vi "Stage Controller.vi"() -> ()   [LabVIEW 2013]
uses:
  <vilib>/Analysis/3filter.llb/Filter Passband Type.ctl
  <userlib>/Agilis Labview 7.1/AGILIS.llb/enter / leave remote mode.vi
  <vilib>/LabVIEW Hacker/LINX/Public/Peripherals/Analog/Analog Read 1 Chan.vi
  <vilib>/LabVIEW Hacker/LINX/LVH-LINX.lvlib
  <vilib>/ptbypt/NI_PtbyPt.lvlib
  <vilib>/Analysis/NI_AALBase.lvlib
panel:
  in  "Move Slide Back":bool
  in  "Move Slide":bool
  in  "Slide Jog Speed":i32(slide) scale=1.0..3.0
  in  "Tab Control":T1(tab)
  out "Main Sig":dbl[][](graph)
  out "Main Output":dbl(graph)
  in  "Arduino Serial Port":refnum<visa-resource-name>="COM3"
  out "Device Name":string
  in  "Analog Channel":u8
  out "Filtered Signal":dbl(graph)
  in  "filter type":T2
  in  "order":i32=2
  in  "initialize":bool
  in  "low cutoff freq: fl":dbl=1.0 format="%#_13g"
  out "Raw Signal":dbl(graph)
  in  "Positive Move Steps":i32=20
  in  "Controller Serial Port":u8=6
  in  "Negative Move Steps":i32=25
  in  "Move Period (ms)":u32=200
  out "Input Signals":dbl[][](graph)
  out "Stepped Signal":dbl(graph)
  in  "Fringe Counter Settings":T3={"Wavelength"=6e-07, "Divisions"=2.0, "Scaling Amplitude"=1.2, "Scaling Offset"=0.0} {"Scaling Offset" format="%0.2f"; "Scaling Amplitude" format="%0.2f"}
  out "Fringe Counter Output Signal":dbl[](graph)
  out "Relative Displacement":dbl=6e-06
  out "Total Displacement":dbl(graph)
  out "Reset Fringe Counter":bool
  out "Displacement":dbl format="%#.3e"
  in  "Motion Direction":bool
  out "stop var":bool
  in  "Move":bool
  out "Timeout":bool
  in  "Error In":errorcluster
  in  "stop":bool
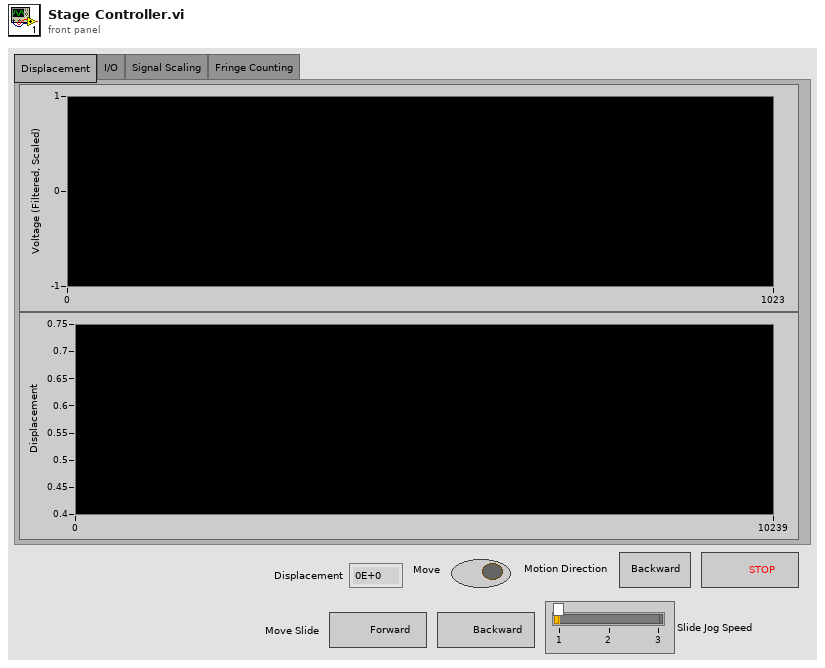
[diagram p1: front panel]
types:
  T1 = enum32{"Displacement", "I/O", "Signal Scaling", "Fringe Counting"}
  T2 = typedef "NI_AALBase.lvlib/Filter Passband Type.ctl" = enum32{"Lowpass", "Highpass", "Bandpass", "Bandstop"}
  T3 = cluster{"Wavelength":dbl, "Divisions":dbl, "Scaling Amplitude":dbl, "Scaling Offset":dbl}
  T4 = typedef "LVH-LINX.lvlib/LINX Ref.ctl" = cluster{"Platform":T5, "Interface":T6, "LINX Device Config":T7}
  T5 = typedef "LVH-LINX.lvlib/Platform.ctl" = enum16{"LINX", "myRIO"}
  T6 = typedef "LVH-LINX.lvlib/Interface.ctl" = enum16{"Serial", "TCP"}
  T7 = typedef "LVH-LINX.lvlib/Device.lvlib/LINX Device Config.ctl" = cluster{"Interface":T6, "COM Port":refnum<visa-resource-name>, "TCP Configuration":T8, "Device Family":T9, "Device ID":u8, "Device Name":string, "TCP Ref":refnum<k5>}
  T8 = typedef "LVH-LINX.lvlib/Device.lvlib/TCP Config.ctl" = cluster{"IP Address":string, "Port":u16}
  T9 = typedef "LVH-LINX.lvlib/Device Family.ctl" = enum8{"National Instruments", "Digilent", "Arduino"}
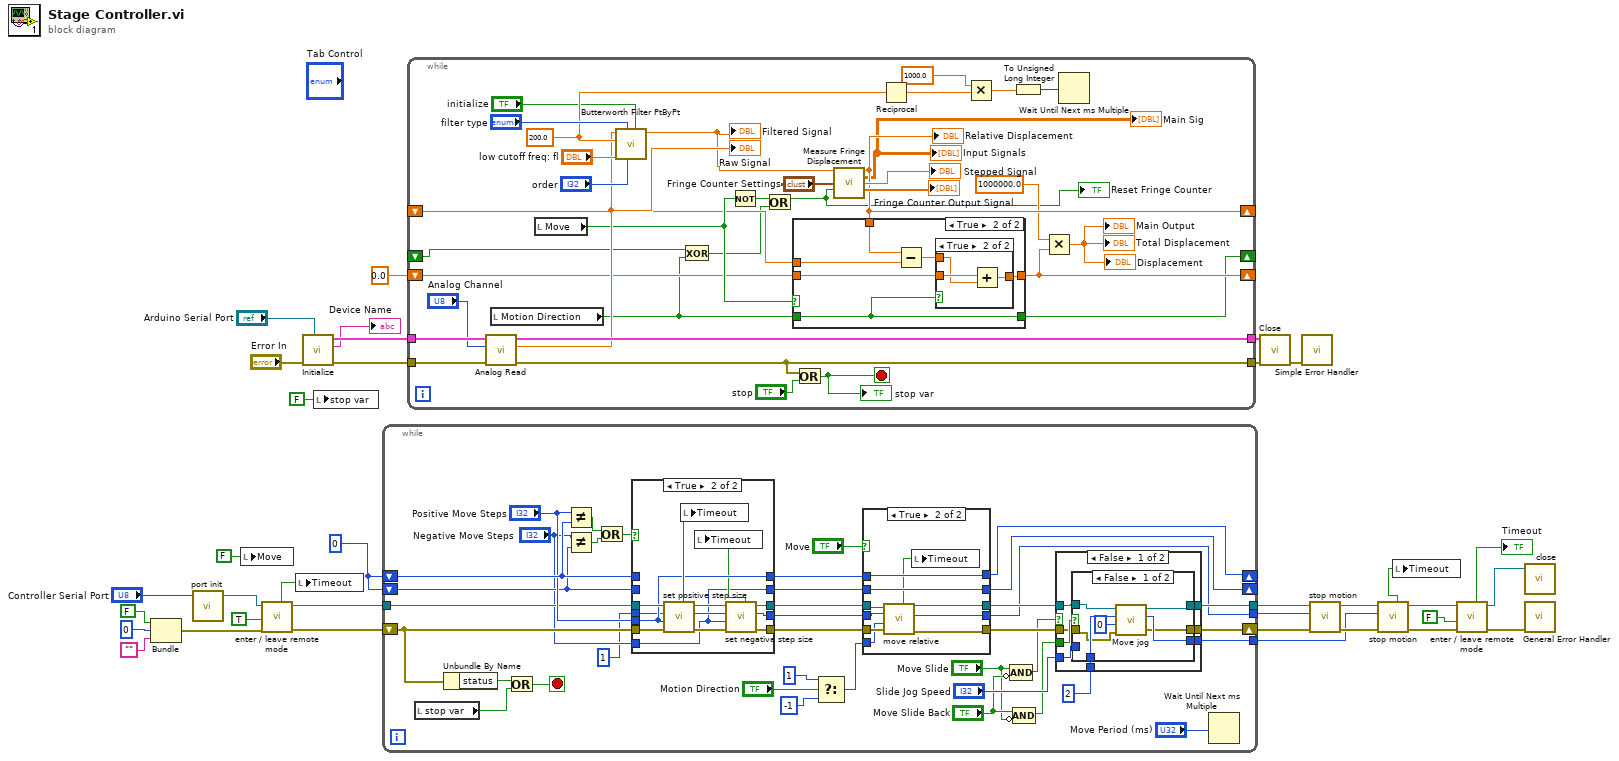
[diagram p0: block diagram]
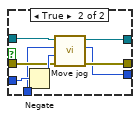
[diagram p2: hidden frame]
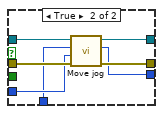
[diagram p3: hidden frame]
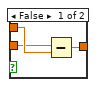
[diagram p7: hidden frame]
diagram:
  w9 = 0
  n1 = Bundle(FALSE, 0, "") -> (w23:errorcluster)  [unwired: 1 in]
  n2 = call <userlib>:"port init.vi"("SerialPort (1)"="Controller Serial Port") -> ("Visa Handle"=w13:refnum<visa-resource-name>)  [unwired: 3 in, 1 out]
  n3 = local write "Move"(FALSE ("Move")) -> ()
  n4 = call "enter / leave remote mode.vi"("error in"=w23, "enter / disable remote mode (True)"=TRUE, "VISA handle in"=w13) -> ("error out"=w20:errorcluster, "VISA handle out"=w21:refnum<visa-resource-name>, "TimeoutFlag"=w22:bool)  [unwired: 6 in]
  n5 = local write "Timeout"(w22) -> ()
  n6 = call <vilib>:"Initialize.vi"("Serial Port"="Arduino Serial Port", "Error In"="Error In") -> ("Error Out"=w32:errorcluster, "Device Name"=→"Device Name":string, "LINX Ref"=w35:T4)  [unwired: 7 in]
  n7 = local write "stop var"(FALSE ("stop var")) -> ()
  n8 = while {
    tunnel: w21 -> [w67]
    shift-right: [w64] -> _
    shift-left: w9 -> [w69]
    shift-right: [w46] -> w5
    shift-left: w20 -> [w72]
    tunnel: [w43] -> w6
    tunnel: [w44] -> w4
    shift-right: [w55] -> _
    shift-left: w9 -> [w54]
    tunnel: [w37] -> w1
    stop <- w71 stop-if-true
    n9 = local read "stop var"() -> (w61:bool)
    n10 = Unbundle By Name(w72) -> ("status"=w70:bool)
    n11 = Or(x=w70, y=w61) -> (x .or. y?=w71:bool)
    n12 = Not Equal?(x="Positive Move Steps", y=w69) -> (x != y?=w73:bool)
    n13 = Not Equal?(x="Negative Move Steps", y=w54) -> (x != y?=w51:bool)
    n14 = Or(x=w73, y=w51) -> (x .or. y?=w52:bool)
    n15 = case shown="True" w52 {
      tunnel: w72 -> [w122 w136]
      tunnel: w67 -> [w121 w134]
      tunnel: 1 ("Axis in") -> [w119 w127]
      tunnel: "Positive Move Steps" -> [_ w128]
      tunnel: [w123 w128] -> w65
      tunnel: w69 -> [w123 _]
      tunnel: [w122 w132] -> w62
      tunnel: [w121 w131] -> w63
      tunnel: "Negative Move Steps" -> [_ w125]
      tunnel: [w120 w125] -> w56
      tunnel: w54 -> [w120 _]
      tunnel: [w119 w124] -> w50
      frame False {
      }
      frame True {
        n16 = call <userlib>:"set positive step size.vi"("error in"=w136, "Step size (positive direction)"=w128, "Axis in"=w127, "VISA Handle in"=w134) -> ("error out"=w133:errorcluster, "Axis out"=w129:i32, "VISA Handle out"=w130:refnum<visa-resource-name>, "TimeoutFlag"=w135:bool)  [unwired: 2 in]
        n17 = local write "Timeout"(w135) -> ()
        n18 = call <userlib>:"set negative step size.vi"("error in"=w133, "Step size (negative direction)"=w125, "Axis in"=w129, "VISA Handle in"=w130) -> ("error out"=w132:errorcluster, "Axis out"=w124:i32, "VISA Handle out"=w131:refnum<visa-resource-name>, "TimeoutFlag"=w126:bool)  [unwired: 2 in]
        n19 = local write "Timeout"(w126) -> ()
      }
    }
    n20 = Select(t=1 ("Number of steps"), s="Motion Direction", f=-1) -> (s? t:f=w58:i32)
    n21 = case shown="True" "Move" {
      tunnel: w65 -> [w108 w114]
      tunnel: [w108 w114] -> w64
      tunnel: w63 -> [w107 w115]
      tunnel: [w107 w116] -> w45
      tunnel: w62 -> [w106 w118]
      tunnel: [w106 w117] -> w47
      tunnel: w58 -> [_ w113]
      tunnel: w56 -> [w105 w112]
      tunnel: [w105 w112] -> w55
      tunnel: [w104 w110] -> w43
      tunnel: w50 -> [w104 w109]
      frame False {
      }
      frame True {
        n22 = call <userlib>:"move relative.vi"("error in"=w118, "Number of steps"=w113, "Axis in"=w109, "VISA Handle in"=w115) -> ("error out"=w117:errorcluster, "Axis out"=w110:i32, "VISA Handle out"=w116:refnum<visa-resource-name>, "TimeoutFlag"=w111:bool)  [unwired: 2 in]
        n23 = local write "Timeout"(w111) -> ()
      }
    }
    n24 = Compound Arithmetic op=AND("Move Slide", invert "Move Slide Back") -> (w41:bool)
    n25 = Compound Arithmetic op=AND("Move Slide Back", invert "Move Slide") -> (w39:bool)
    n26 = case shown="False" w41 {
      tunnel: w47 -> [w79 w103]
      tunnel: [w78 w102] -> w46
      tunnel: w45 -> [w77 w101]
      tunnel: [w76 w100] -> w44
      tunnel: "Slide Jog Speed" -> [w81 w99]
      tunnel: w39 -> [w80 _]
      tunnel: [w74 w98] -> w37
      tunnel: u32 2 ("Axis in") -> [w75 w97]
      frame False {
        n27 = case shown="False" w80 {
          tunnel: w81 -> [_ w96]
          tunnel: w79 -> [w82 w94]
          tunnel: [w83 w93] -> w78
          tunnel: w77 -> [w85 w92]
          tunnel: [w84 w91] -> w76
          tunnel: w75 -> [w88 w90]
          tunnel: [w86 w89] -> w74
          frame False {
            n28 = call <userlib>:"Move jog.vi"("error in"=w82, "Jog mode"=0, "Axis in"=w88, "VISA Handle in"=w85) -> ("error out"=w83:errorcluster, "Axis out"=w86:i32, "VISA Handle out"=w84:refnum<visa-resource-name>)  [unwired: 2 in, 1 out]
          }
          frame True {
            n29 = Negate(x=w96) -> (-x=w95:i32)
            n30 = call <userlib>:"Move jog.vi"("error in"=w94, "Jog mode"=w95, "Axis in"=w90, "VISA Handle in"=w92) -> ("error out"=w93:errorcluster, "Axis out"=w89:i32, "VISA Handle out"=w91:refnum<visa-resource-name>)  [unwired: 2 in, 1 out]
          }
        }
      }
      frame True {
        n31 = call <userlib>:"Move jog.vi"("error in"=w103, "Jog mode"=w99, "Axis in"=w97, "VISA Handle in"=w101) -> ("error out"=w102:errorcluster, "Axis out"=w98:i32, "VISA Handle out"=w100:refnum<visa-resource-name>)  [unwired: 2 in, 1 out]
      }
    }
    n32 = Wait Until Next ms Multiple(millisecond multiple="Move Period (ms)") -> ()  [unwired: 1 out]
  }
  n33 = while {
    tunnel: w35 -> [w171]
    tunnel: [w170] -> w34
    tunnel: [w165] -> w33
    tunnel: w32 -> [w169]
    shift-right: [w146] -> _
    shift-left: 0.0 ("Displacement") -> [w149]
    shift-right: [w147] -> _
    shift-left: _ -> [w148]
    shift-right: [w141] -> _
    shift-left: _ -> [w138]
    stop <- w166 stop-if-true
    w162 = 200.0 ("sampling freq: fs")
    n34 = call-poly <vilib>:"Analog Read.vi"("Error In"=w169, "Analog Channel"="Analog Channel", "LINX Resource"=w171) -> ("Error Out"=w165:errorcluster, "AI Value"=w155:dbl, "LINX Resource"=w170:T4)  [unwired: 5 in, 1 out]
    "Raw Signal" <- w155
    n35 = local read "Motion Direction"() -> (w137:bool)
    n36 = local read "Move"() -> (w150:bool)
    n37 = call <vilib>:"Butterworth Filter PtByPt.vi"("initialize"="initialize", "order"="order", "filter type"="filter type", "low cutoff freq: fl"="low cutoff freq: fl", "sampling freq: fs"=w162, "x"=w155) -> ("Filtered x"=w143:dbl)  [unwired: 3 in, 1 out]
    "Filtered Signal" <- w143
    n38 = Exclusive Or(1:w137, 2:w138) -> (0:w139:bool)
    n39 = Not(x=w150) -> (.not. x?=w151:bool)
    n40 = Or(x=w151, y=w139) -> (x .or. y?=w140:bool)
    "Reset Fringe Counter" <- w140
    n41 = Or(x=w165, y="stop") -> (x .or. y?=w166:bool)
    "stop var" <- w166
    n42 = call "Measure Fringe Displacement.vi"("Photodiode Output"=w143, "Fringe Counter Settings"="Fringe Counter Settings", "Reset"=w140) -> ("Displacement"=w147:dbl, "Input Signals"=→"Input Signals" →"Main Sig":dbl[][], "Stepped Signal"=→"Stepped Signal":dbl, "Output Signal"=→"Fringe Counter Output Signal":dbl[])  [unwired: 8 in, 1 out]
    "Relative Displacement" <- w147
    n43 = case shown="True" w150 {
      tunnel: w149 -> [w173 w178]
      tunnel: [w173 w179] -> w146
      tunnel: w148 -> [_ w177]
      tunnel: w147 -> [_ w175]
      tunnel: w137 -> [w172 w174]
      tunnel: [w172 w174] -> w141
      frame False {
      }
      frame True {
        n44 = Subtract(x=w175, y=w177) -> (x-y=w176:dbl)
        n45 = case shown="True" w174 {
          tunnel: [w182 w185] -> w179
          tunnel: w178 -> [w180 w184]
          tunnel: w176 -> [w181 w183]
          frame False {
            n46 = Subtract(x=w180, y=w181) -> (x-y=w182:dbl)
          }
          frame True {
            n47 = Add(x=w184, y=w183) -> (x+y=w185:dbl)
          }
        }
      }
    }
    n48 = Reciprocal(x=w162) -> (1/x=w160:dbl)
    n49 = Multiply(x=1000.0 ("y"), y=w160) -> (x*y=w159:dbl)
    n50 = To Unsigned Long Integer(number=w159) -> (unsigned 32bit integer=w158:u32)
    n51 = Multiply(x=1000000.0, y=w146) -> (x*y=→"Displacement" →"Total Displacement" →"Main Output":dbl)
    n52 = Wait Until Next ms Multiple(millisecond multiple=w158) -> ()  [unwired: 1 out]
  }
  n53 = call <vilib>:"Close.vi"("Error In"=w33, "LINX Resource"=w34) -> ("Error Out"=w29:errorcluster)  [unwired: 8 in, 1 out]
  n54 = call <vilib>:"Simple Error Handler.vi"("error in (no error)"=w29) -> ()  [unwired: 4 in, 5 out]
  n55 = call <userlib>:"stop motion.vi"("error in"=w5, "Axis in"=w6, "VISA Handle in"=w4) -> ("error out"=w3:errorcluster, "VISA Handle out"=w2:refnum<visa-resource-name>)  [unwired: 3 in, 2 out]
  n56 = call <userlib>:"stop motion.vi"("error in"=w3, "Axis in"=w1, "VISA Handle in"=w2) -> ("error out"=w19:errorcluster, "VISA Handle out"=w12:refnum<visa-resource-name>, "TimeoutFlag"=w16:bool)  [unwired: 3 in, 1 out]
  n57 = local write "Timeout"(w16) -> ()
  n58 = call "enter / leave remote mode.vi"("error in"=w19, "enter / disable remote mode (True)"=FALSE, "VISA handle in"=w12) -> ("error out"=w15:errorcluster, "VISA handle out"=w14:refnum<visa-resource-name>, "TimeoutFlag"=→"Timeout":bool)  [unwired: 6 in]
  n59 = call <vilib>:"close.vi"("VISA Handle in"=w14) -> ()  [unwired: 4 in, 1 out]
  n60 = call <vilib>:"General Error Handler.vi"("error in (no error)"=w15) -> ()  [unwired: 10 in, 5 out]
